vi "Read Output (Multiple).vi"(8 "error in (no error)":errorcluster, 10 "Channel (1: Channel 1)":i32(ring)=1 items=["Channel 1"=1, "Channel 2"=2, "Channel 3"=3], 11 "VISA resource name":refnum<visa-resource-name>) -> (0 "error out":errorcluster, 1 "Actual Current Level (A)":dbl[](array[numeric]) format="%.2g", 2 "Actual Voltage Level (V)":dbl[](array[numeric]) format="%.2g", 3 "VISA resource name out":refnum<visa-resource-name>)   [LabVIEW 2018, in "Agilent U2722.lvlib"]
doc: "Returns the actual voltage level and actual current level for a desired channel."
uses:
  Agilent U2722.lvlib
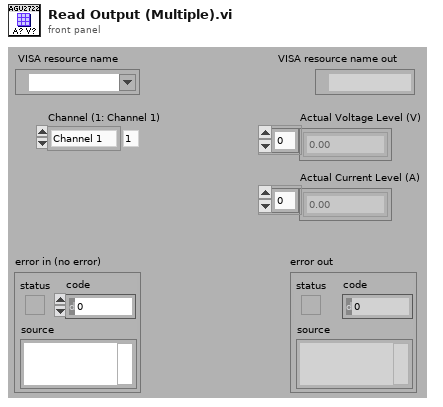
[diagram p1: front panel]
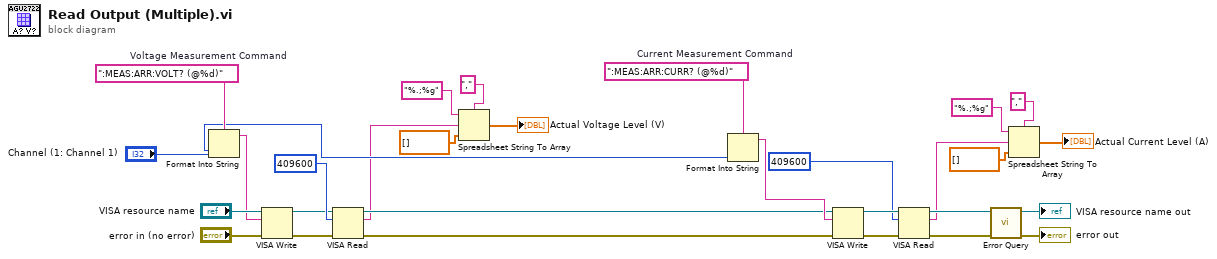
[diagram p0: block diagram]
diagram:
  w19 = ":MEAS:ARR:CURR? (@%d)"  # Current Measurement Command
  w20 = ":MEAS:ARR:VOLT? (@%d)"  # Voltage Measurement Command
  n1 = Format Into String(format string=w20, "Channel (1: Channel 1)") -> (resulting string=w17:string)  [unwired: 2 in, 1 out]
  n2 = VISA Write(VISA resource name="VISA resource name", write buffer=w17, error in (no error)="error in (no error)") -> (VISA resource name out=w15:refnum<visa-resource-name>, error out=w14:errorcluster)  [unwired: 1 out]
  n3 = VISA Read(VISA resource name=w15, byte count=u32 409600, error in (no error)=w14) -> (VISA resource name out=w11:refnum<visa-resource-name>, read buffer=w8:string, error out=w23:errorcluster)  [unwired: 1 out]
  n4 = Spreadsheet String To Array(delimiter (Tab)=",", format string="%.;%g", spreadsheet string=w8, array type (2D Dbl)=dbl[] []) -> (array=→"Actual Voltage Level (V)":dbl[])
  n5 = Format Into String(format string=w19, "Channel (1: Channel 1)") -> (resulting string=w12:string)  [unwired: 2 in, 1 out]
  n6 = VISA Write(VISA resource name=w11, write buffer=w12, error in (no error)=w23) -> (VISA resource name out=w27:refnum<visa-resource-name>, error out=w26:errorcluster)  [unwired: 1 out]
  n7 = VISA Read(VISA resource name=w27, byte count=u32 409600, error in (no error)=w26) -> (VISA resource name out=w25:refnum<visa-resource-name>, read buffer=w2:string, error out=w24:errorcluster)  [unwired: 1 out]
  n8 = call "Error Query.vi"("error in (no error)"=w24, "VISA resource name"=w25) -> ("error out"=→"error out":errorcluster, "VISA resource name out"=→"VISA resource name out":refnum<visa-resource-name>)  [unwired: 6 in, 2 out]
  n9 = Spreadsheet String To Array(delimiter (Tab)=",", format string="%.;%g", spreadsheet string=w2, array type (2D Dbl)=dbl[] []) -> (array=→"Actual Current Level (A)":dbl[])
